vi "test - NESTED read.vi"(8 "error in (no error)":errorcluster, 11 "TestCase in":refnum<class "csm-ini-variable-addon.lvclass">) -> (0 "error out":errorcluster, 3 "TestCase out":refnum<class "csm-ini-variable-addon.lvclass">)   [LabVIEW 2017, in "csm-ini-variable-addon.lvclass"]
uses:
  csm-ini-variable-addon.lvclass
  51eeedc8-b31c-488c-8392-a86325f3fef9.vi
  d661d301-294d-4a40-9fe1-44519e1c8482.vi
  394c0a32-ea4a-4895-9acd-42f6254c3441.vi
  51eeedc8-b31c-488c-8392-a86325f3fef9.vi/b09b9099-6be0-413b-8afc-4908471460c3.vi
  d661d301-294d-4a40-9fe1-44519e1c8482.vi/b09b9099-6be0-413b-8afc-4908471460c3.vi
  394c0a32-ea4a-4895-9acd-42f6254c3441.vi/b09b9099-6be0-413b-8afc-4908471460c3.vi
  INI-Static-Variable-Support/_Support/global-csm-ini-db-change-flag.vi
  <vilib>/Utility/Data Type/Get Type Information.vi
  <userlib>/_NEVSTOP/Communicable State Machine(CSM)/addons/API-String-Arugments-Support/_Support/Data To SingleElementsArray_csm.vi
  INI-Static-Variable-Support/_Support/Parse Used Session and Name.vi
  <userlib>/_NEVSTOP/Communicable State Machine(CSM)/addons/API-String-Arugments-Support/_Support/Data To API String Arguments.vi
  INI-Static-Variable-Support/_Support/INI-FGV(lvlibp).vi
  INI-Static-Variable-Support/_Support/Populate String with INI Variable.vi
  <userlib>/_NEVSTOP/Communicable State Machine(CSM)/addons/API-String-Arugments-Support/_Support/Convert API String Arguments to Data(variant).vi
  <userlib>/_NEVSTOP/Communicable State Machine(CSM)/addons/API-String-Arugments-Support/_Support/SingleElementsArray To Data_csm.vi
  INI-Static-Variable-Support/INI-Static-Variable-Support.lvlib
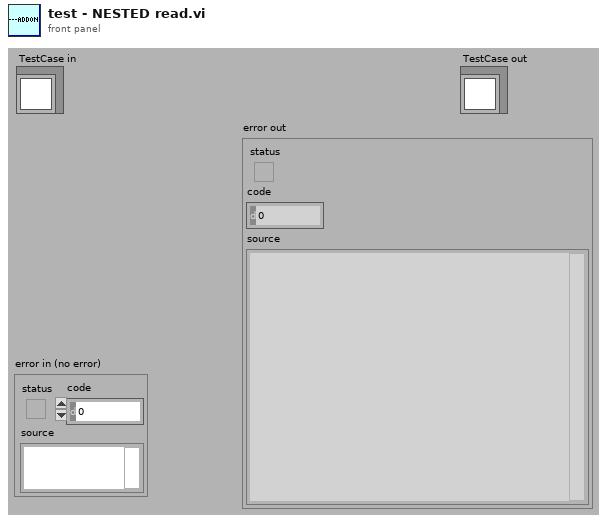
[diagram p1: front panel]
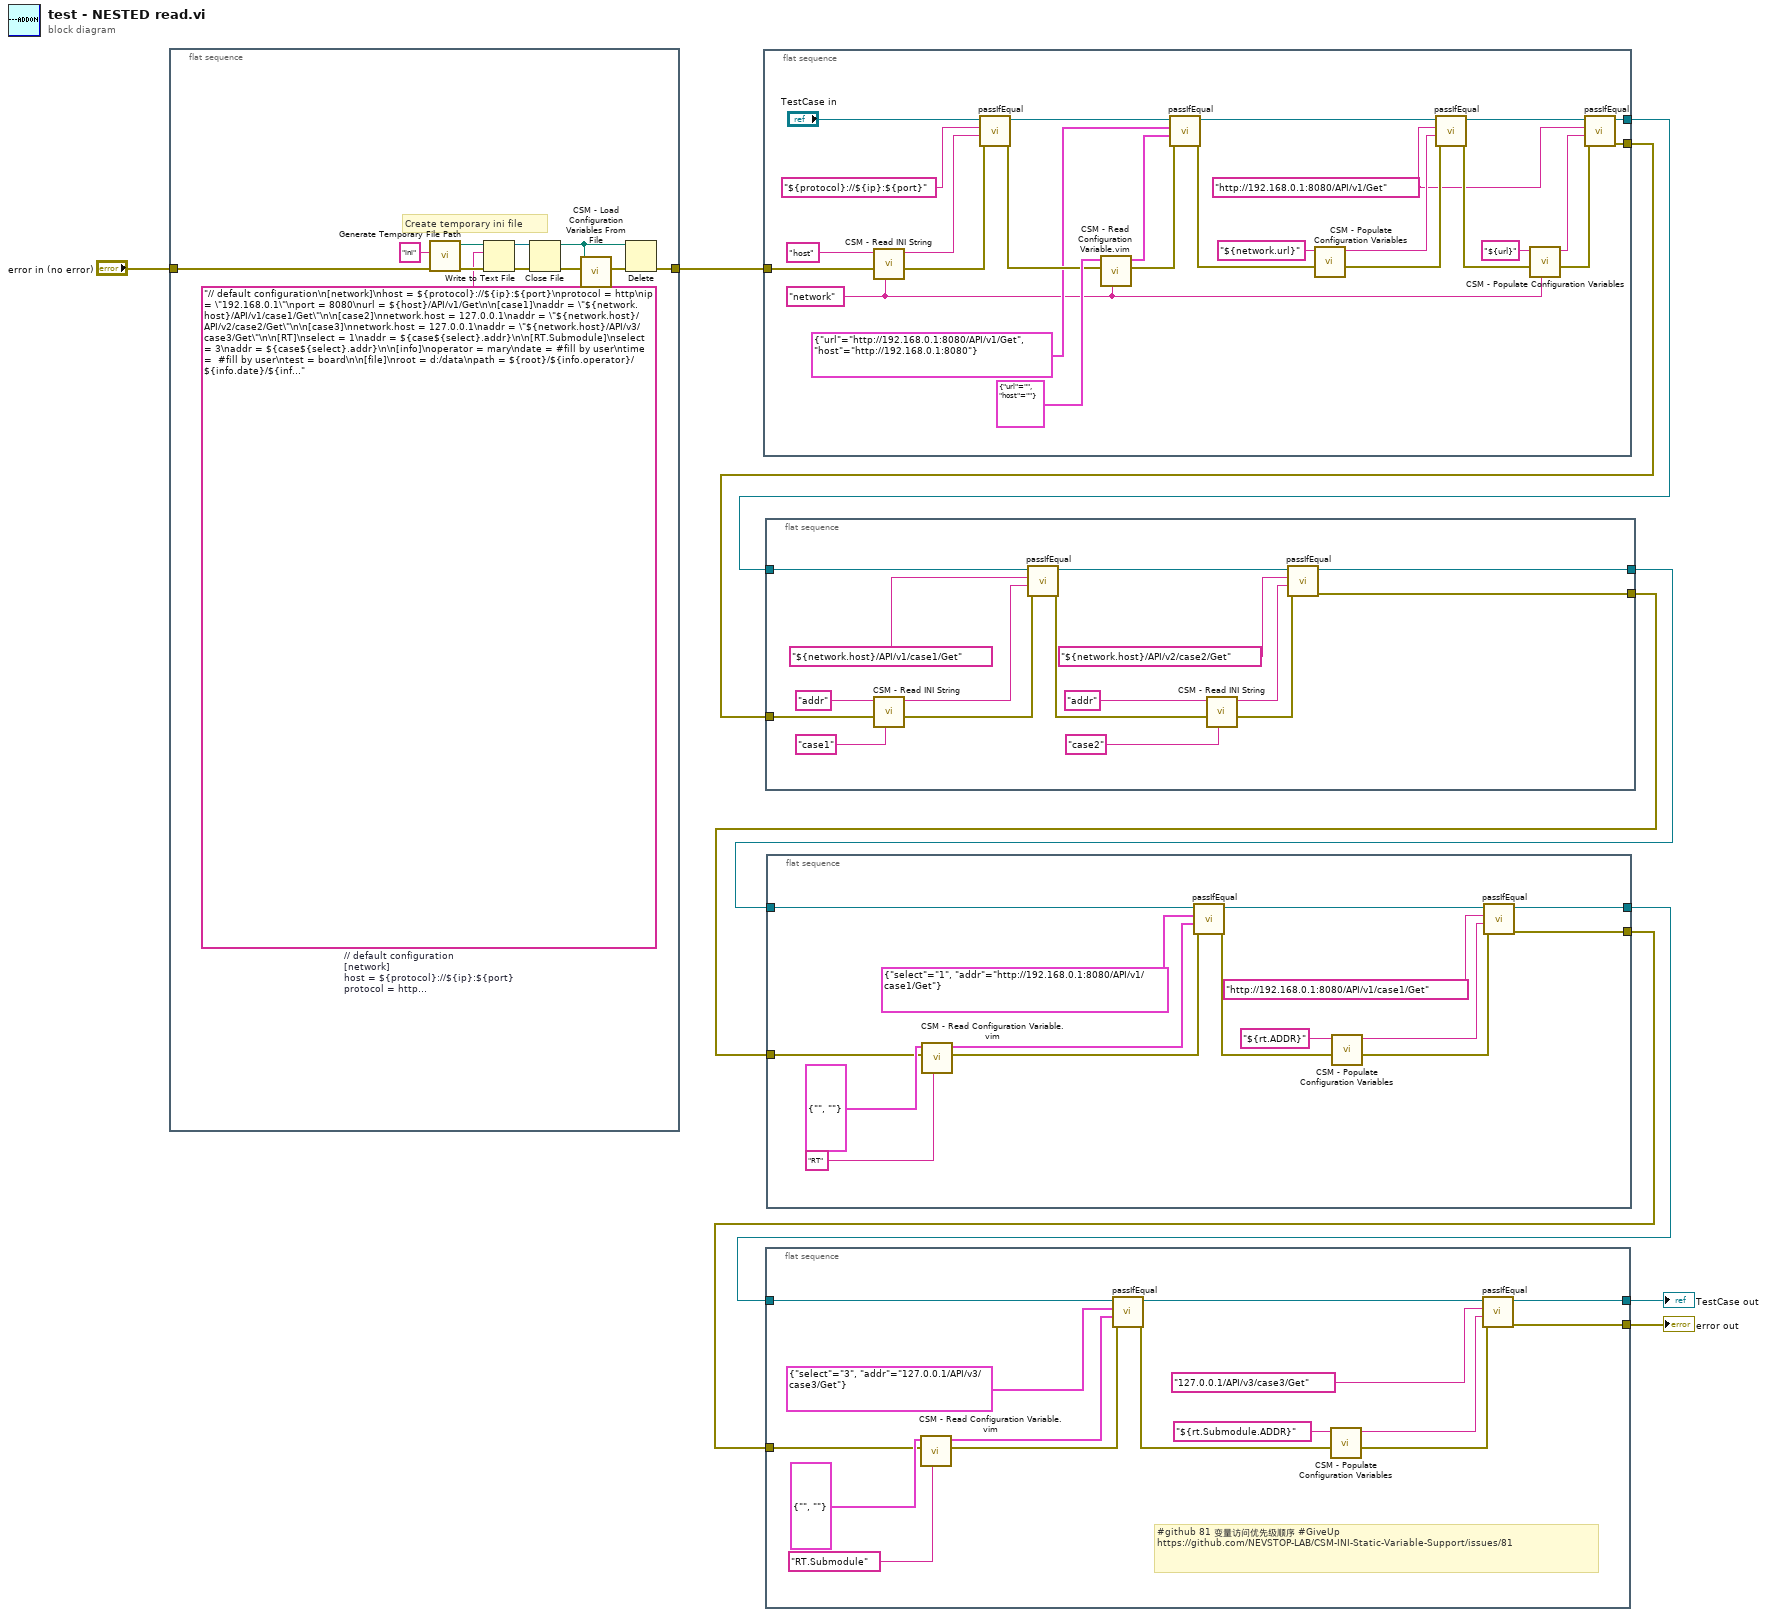
[diagram p0: block diagram]
diagram:
  n1 = flat-sequence {
    tunnel: "error in (no error)" -> [w21]
    tunnel: [w20] -> w9
    frame #0 {
      w13 = "// default configuration\n[network]\nhost = ${protocol}://${ip}:${port}\nprotocol = http\nip = \"192.168.0.1\"\nport = 8080\nurl = ${host}/API/v1/Get\n\n[case1]\naddr = \"${network.host}/API/v1/case1/Get\"\n\n[case2]\nnetwork.host = 127.0.0.1\naddr = \"${network.host}/API/v2/case2/Get\"\n\n[case3]\nnetwork.host = 127.0.0.1\naddr = \"${network.host}/API/v3/case3/Get\"\n\n[RT]\nselect = 1\naddr = ${case${select}.addr}\n\n[RT.Submodule]\nselect = 3\naddr = ${case${select}.addr}\n\n[info]\noperator = mary\ndate = #fill by user\ntime =  #fill by user\ntest = board\n\n[file]\nroot = d:/data\npath = ${root}/${info.operator}/${info.date}/${info.test}${info.time}.tdms"  # // default configuration [network] host = ${protocol}://${ip}:${port} protocol = http ip = "192.168.0.1" port = 8080 url = ${host}/API/v1/Get  [case1] addr = "${network.host}/API/v1/case1/Get"  [case2] network.host = 127.0.0.1 addr = "${network.host}/API/v2/case2/Get"  [case3] network.host = 127.0.0.1 addr = "${network.host}/API/v3/case3/Get"  [RT] select = 1 addr = ${case${select}.addr}  [RT.Submodule] select = 3 addr = ${case${select}.addr}  [info] operator = mary date = #fill by user time =  #fill by user test = board  [file] root = d:/data path = ${root}/${info.operator}/${info.date}/${info.test}${info.time}.tdms
      # "Create temporary ini file"
      n2 = call <vilib>:"Generate Temporary File Path.vi"("error in (no error)"=w21, "Temporary File Extension (tmp)"="ini") -> ("error out"=w19:errorcluster, "Unique Temporary File Path"=w16:path)  [unwired: 8 in]
      n3 = Write to Text File(file (use dialog)=w16, text=w13, error in=w19) -> (refnum out=w15:refnum<file>, error out=w17:errorcluster)  [unwired: 1 in, 1 out]
      n4 = Close File(refnum=w15, error in=w17) -> (path=w11:path, error out=w14:errorcluster)
      n5 = call "CSM - Load Configuration Variables From File.vi"("error in (no error)"=w14, "Path"=w11) -> ("error out"=w12:errorcluster)  [unwired: 7 in]
      n6 = Delete(path (use dialog)=w11, error in=w12) -> (error out=w20:errorcluster)  [unwired: 3 in, 2 out]
    }
  }
  n7 = flat-sequence {
    tunnel: w9 -> [w47]
    tunnel: [w23] -> w8
    tunnel: [w22] -> w7
    frame #0 {
      w26 = "http://192.168.0.1:8080/API/v1/Get" ("${network.url}")
      w29 = "network" ("Section Name(\"\" as Default)")
      n8 = call "CSM - Read INI String.vi"("Section Name(\"\" as Default)"=w29, "error in (no error)"=w47, "String in"="host") -> ("error out"=w44:errorcluster, "String out"=w45:string)  [unwired: 4 in, 1 out]
      n9 = call-dynamic "passIfEqual.vi"("error in (no error)"=w44, "y"=w45, "x"="${protocol}://${ip}:${port}" ("String in"), "TestCase in"="TestCase in") -> ("error out"=w41:errorcluster, "TestCase out"=w39:refnum<class "csm-ini-variable-addon.lvclass">)  [unwired: 6 in]
      n10 = call "CSM - Read Configuration Variable.vim"("Section Name(\"\" as Default)"=w29, "error in (no error)"=w41, "config prototype(Cluster Prefered)"=cluster{"url":string, "host":string} {"url"="", "host"=""}) -> ("error out"=w40:errorcluster, "config out"=w38:cluster{"url":string, "host":string})  [unwired: 5 in]
      n11 = call-dynamic "passIfEqual.vi"("error in (no error)"=w40, "y"=w38, "x"=cluster{"url":string, "host":string} {"url"="http://192.168.0.1:8080/API/v1/Get", "host"="http://192.168.0.1:8080"} ("network.cluster"), "TestCase in"=w39) -> ("error out"=w34:errorcluster, "TestCase out"=w33:refnum<class "csm-ini-variable-addon.lvclass">)  [unwired: 6 in]
      n12 = call "CSM - Populate Configuration Variables.vi"("error in (no error)"=w34, "String in"="${network.url}") -> ("error out"=w31:errorcluster, "String out"=w32:string)  [unwired: 6 in]
      n13 = call-dynamic "passIfEqual.vi"("error in (no error)"=w31, "y"=w32, "x"=w26, "TestCase in"=w33) -> ("error out"=w30:errorcluster, "TestCase out"=w28:refnum<class "csm-ini-variable-addon.lvclass">)  [unwired: 6 in]
      n14 = call "CSM - Populate Configuration Variables.vi"("Section Name(\"\" as Default)"=w29, "error in (no error)"=w30, "String in"="${url}") -> ("error out"=w27:errorcluster, "String out"=w25:string)  [unwired: 5 in]
      n15 = call-dynamic "passIfEqual.vi"("error in (no error)"=w27, "y"=w25, "x"=w26, "TestCase in"=w28) -> ("error out"=w22:errorcluster, "TestCase out"=w23:refnum<class "csm-ini-variable-addon.lvclass">)  [unwired: 6 in]
    }
  }
  n16 = flat-sequence {
    tunnel: w8 -> [w51]
    tunnel: w7 -> [w50]
    tunnel: [w49] -> w6
    tunnel: [w48] -> w5
    frame #0 {
      n17 = call "CSM - Read INI String.vi"("Section Name(\"\" as Default)"="case1" ("Section Name(\"\" as Default)"), "error in (no error)"=w50, "String in"="addr") -> ("error out"=w59:errorcluster, "String out"=w60:string)  [unwired: 4 in, 1 out]
      n18 = call-dynamic "passIfEqual.vi"("error in (no error)"=w59, "y"=w60, "x"="${network.host}/API/v1/case1/Get" ("case1.addr"), "TestCase in"=w51) -> ("error out"=w58:errorcluster, "TestCase out"=w61:refnum<class "csm-ini-variable-addon.lvclass">)  [unwired: 6 in]
      n19 = call "CSM - Read INI String.vi"("Section Name(\"\" as Default)"="case2" ("Section Name(\"\" as Default)"), "error in (no error)"=w58, "String in"="addr") -> ("error out"=w62:errorcluster, "String out"=w63:string)  [unwired: 4 in, 1 out]
      n20 = call-dynamic "passIfEqual.vi"("error in (no error)"=w62, "y"=w63, "x"="${network.host}/API/v2/case2/Get" ("case2.addr"), "TestCase in"=w61) -> ("error out"=w48:errorcluster, "TestCase out"=w49:refnum<class "csm-ini-variable-addon.lvclass">)  [unwired: 6 in]
    }
  }
  n21 = flat-sequence {
    tunnel: w4 -> [w67]
    tunnel: w3 -> [w66]
    tunnel: [w65] -> w2
    tunnel: [w64] -> w1
    frame #0 {
      # "#github 81 变量访问优先级顺序 #GiveUp\nhttps://github.com/NEVSTOP-LAB/CSM-INI-Static-Variable-Support/issues/81"
      n22 = call "CSM - Read Configuration Variable.vim"("Section Name(\"\" as Default)"="RT.Submodule" ("Section Name(\"\" as Default)"), "error in (no error)"=w66, "config prototype(Cluster Prefered)"=cluster{"select":string, "addr":string} {"select"="", "addr"=""}) -> ("error out"=w73:errorcluster, "config out"=w74:cluster{"select":string, "addr":string})  [unwired: 5 in]
      n23 = call-dynamic "passIfEqual.vi"("error in (no error)"=w73, "y"=w74, "x"=cluster{"select":string, "addr":string} {"select"="3", "addr"="127.0.0.1/API/v3/case3/Get"} ("rt.cluster"), "TestCase in"=w67) -> ("error out"=w75:errorcluster, "TestCase out"=w76:refnum<class "csm-ini-variable-addon.lvclass">)  [unwired: 6 in]
      n24 = call "CSM - Populate Configuration Variables.vi"("error in (no error)"=w75, "String in"="${rt.Submodule.ADDR}") -> ("error out"=w77:errorcluster, "String out"=w78:string)  [unwired: 6 in]
      n25 = call-dynamic "passIfEqual.vi"("error in (no error)"=w77, "y"=w78, "x"="127.0.0.1/API/v3/case3/Get" ("${rt.addr}"), "TestCase in"=w76) -> ("error out"=w64:errorcluster, "TestCase out"=w65:refnum<class "csm-ini-variable-addon.lvclass">)  [unwired: 6 in]
    }
  }
  n26 = flat-sequence {
    tunnel: w6 -> [w82]
    tunnel: w5 -> [w81]
    tunnel: [w80] -> w4
    tunnel: [w79] -> w3
    frame #0 {
      n27 = call "CSM - Read Configuration Variable.vim"("Section Name(\"\" as Default)"="RT" ("Section Name(\"\" as Default)"), "error in (no error)"=w81, "config prototype(Cluster Prefered)"=cluster{"select":string, "addr":string} {"select"="", "addr"=""}) -> ("error out"=w88:errorcluster, "config out"=w89:cluster{"select":string, "addr":string})  [unwired: 5 in]
      n28 = call-dynamic "passIfEqual.vi"("error in (no error)"=w88, "y"=w89, "x"=cluster{"select":string, "addr":string} {"select"="1", "addr"="http://192.168.0.1:8080/API/v1/case1/Get"} ("rt.cluster"), "TestCase in"=w82) -> ("error out"=w90:errorcluster, "TestCase out"=w91:refnum<class "csm-ini-variable-addon.lvclass">)  [unwired: 6 in]
      n29 = call "CSM - Populate Configuration Variables.vi"("error in (no error)"=w90, "String in"="${rt.ADDR}") -> ("error out"=w92:errorcluster, "String out"=w93:string)  [unwired: 6 in]
      n30 = call-dynamic "passIfEqual.vi"("error in (no error)"=w92, "y"=w93, "x"="http://192.168.0.1:8080/API/v1/case1/Get" ("${rt.addr}"), "TestCase in"=w91) -> ("error out"=w79:errorcluster, "TestCase out"=w80:refnum<class "csm-ini-variable-addon.lvclass">)  [unwired: 6 in]
    }
  }
  "error out" <- w1
  "TestCase out" <- w2
